vi "time-sec-to-time-str.vi"(1 "Numeric":dbl format="%_6g") -> (0 "formatted-str":string)   [LabVIEW 2010]
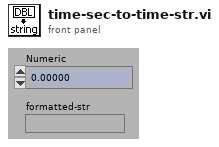
[diagram p1: front panel]
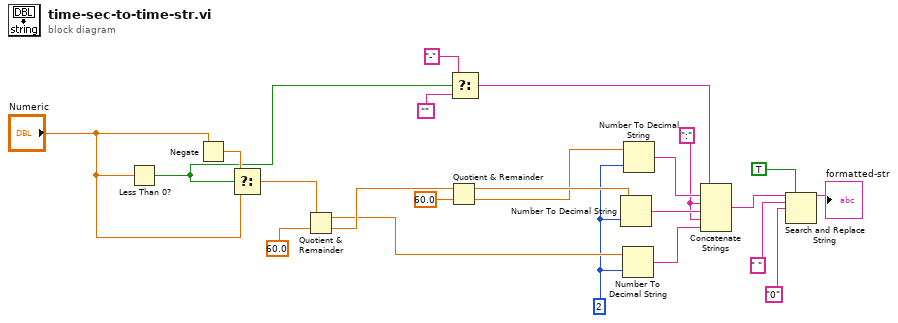
[diagram p0: block diagram]
diagram:
  w1 = i16 2 ("width (-)")
  w14 = ":" ("string")
  n1 = Less Than 0?(x="Numeric") -> (x < 0?=w6:bool)
  n2 = Negate(x="Numeric") -> (-x=w9:dbl)
  n3 = Select(t=w9, s=w6, f="Numeric") -> (s? t:f=w8:dbl)
  n4 = Quotient & Remainder(x=w8, y=60.0) -> (x-y*floor(x/y)=w11:dbl, floor(x/y)=w13:dbl)
  n5 = Quotient & Remainder(x=w13, y=60.0) -> (x-y*floor(x/y)=w10:dbl, floor(x/y)=w5:dbl)
  n6 = Select(t="-" ("string"), s=w6, f="") -> (s? t:f=w4:string)
  n7 = Number To Decimal String(number=w10, width (-)=w1) -> (decimal integer string=w20:string)
  n8 = Number To Decimal String(number=w11, width (-)=w1) -> (decimal integer string=w19:string)
  n9 = Number To Decimal String(number=w5, width (-)=w1) -> (decimal integer string=w21:string)
  n10 = Concatenate Strings(w4, w21, w14, w20, w14, w19) -> (w18:string)
  n11 = Search and Replace String(replace all?=TRUE ("replace all? (F)"), input string=w18, search string=" ", replace string="0" ("replace string (\"\")")) -> (result string=→"formatted-str":string)  [unwired: 4 in, 3 out]
